vi "Get All Supported DataRates.vi"(8 "error in (no error)":errorcluster, 11 "TLCamera reference":refnum<k24>) -> (0 "error out":errorcluster, 2 "Supported DataRates":i32[](array[numeric]), 3 "TLCamera reference out":refnum<k24>)   [LabVIEW 2015]
uses:
  C:/code/Host/Installer/Scientific Camera Interfaces/LabVIEW/32_bit/Library_X86/Thorlabs.TSI.TLCameraInterfaces.dll
  code/Host/Installer/Scientific Camera Interfaces/LabVIEW/32_bit/Library_X86/Thorlabs.TSI.TLCameraInterfaces.dll
panel:
  in  "Data Rate":i32(ring) items=["ReadoutSpeed20MHz", "ReadoutSpeed40MHz", "FPS30", "FPS50"]
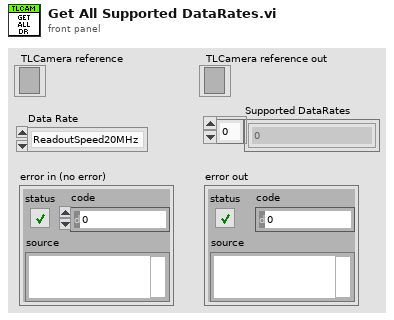
[diagram p1: front panel]
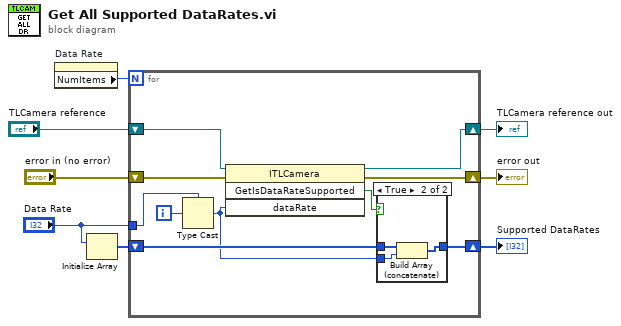
[diagram p0: block diagram]
diagram:
  n1 = property on="Data Rate" class="Ring (strict)"() -> ("NumItems"=w8:u32)  [unwired: 2 in, 2 out]
  n2 = Initialize Array("Data Rate") -> (w4:i32[])  [unwired: 1 in]
  n3 = for {
    N: w8 -> [_]
    shift-right: [w9] -> w3
    shift-left: "error in (no error)" -> [w17]
    tunnel: "Data Rate" -> [w14]
    shift-right: [w11] -> w1
    shift-left: w4 -> [w13]
    shift-right: [w10] -> w2
    shift-left: "TLCamera reference" -> [w18]
    i -> [w16]
    n4 = Type Cast(type=w14, x=w16) -> (*(type *) &x=w12:i32)
    n5 = invoke class="ITLCamera" method="GetIsDataRateSupported"(reference=w18, error in=w17, "dataRate"=w12) -> (reference out=w10:refnum<k24>, error out=w9:errorcluster, "GetIsDataRateSupported"=w15:bool)  [unwired: 1 in, 1 out]
    n6 = case shown="True" w15 {
      tunnel: w13 -> [w19 w22]
      tunnel: w12 -> [_ w21]
      tunnel: [w19 w20] -> w11
      frame False {
      }
      frame True {
        n7 = Build Array (concatenate)(w22, w21) -> (w20:i32[])
      }
    }
  }
  "error out" <- w3
  "TLCamera reference out" <- w2
  "Supported DataRates" <- w1
